vi "FilePath.vi"() -> ()   [LabVIEW 2020]
panel:
  in  "Path":path
  # "Path to CommandTemplates folder"
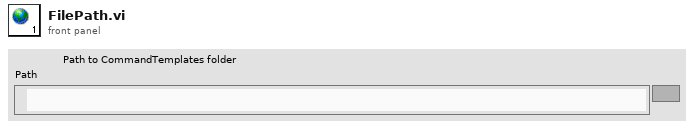
[diagram p1: front panel]
diagram:
